vi "Read Offline Data.vi"(8 "Error In":errorcluster) -> (0 "Error Out":errorcluster)   [LabVIEW 2014, in "Aquisicao de Dados.lvlib"]
uses:
  Aquisicao de Dados.lvlib
  <vilib>/Waveform/WDTOps.llb/WDT Waveform Duration DBL.vi
  <vilib>/Waveform/WDTOps.llb/WDT Number of Waveform Samples DBL.vi
  <vilib>/measure/mascope.llb/Amplitude and Levels 1 chan.vi
  <vilib>/Waveform/WDTOps.llb/WDT Get Waveform Subset DBL.vi
  <vilib>/express/express analysis/Spectral/Block/exnSpectralBlock spectral measurements peak poly.vi
  <vilib>/express/express analysis/Spectral/Block/exnSpectralBlock spectral measurements peak WFM.vi
  <vilib>/express/express analysis/Spectral/XNode/ExpressSpectralMeasurementsBlockNode.xnode
  <vilib>/measure/NI_MAPro.lvlib
panel:
  out "Espectro Janelado":cluster{"f0":dbl, "df":dbl, "magnitude":dbl[]}(graph)
  in  "Duração":dbl(slide) scale=0.0..5.0
  in  "T inicial":dbl(slide) scale=0.0..5.0
  out "Frequência Fundamental":dbl
  out "Mulher":bool
  out "Homem":bool
  out "Canal 0":waveform(dbl)(graph)
  out "Resolução de Frequência":dbl
  out "Frequência Associada":dbl
  out "Maior Amplitude":dbl
  out "Período Amostral (s)":dbl
  out "Frequência Amostral (Hz)":dbl
  out "Número Amostral":dbl
  out "Amplitude do Sinal (%)":dbl
  out "Espectro do Canal 0":cluster{"f0":dbl, "df":dbl, "magnitude":dbl[]}(graph)
  out "Espectro do Canal 1":cluster{"f0":dbl, "df":dbl, "magnitude":dbl[]}(graph)
  out "Resolução de Frequência":dbl
  out "Frequência Associada":dbl
  out "Maior Amplitude":dbl
  out "Período Amostral (s)":dbl
  out "Frequência Amostral (Hz)":dbl
  out "Número Amostral":dbl
  out "Amplitude do Sinal (%)":dbl
  out "Canal 1":waveform(dbl)(graph)
  # "Dados do Sinal do Canal 0"
  # "Dados do Sinal do Canal 1"
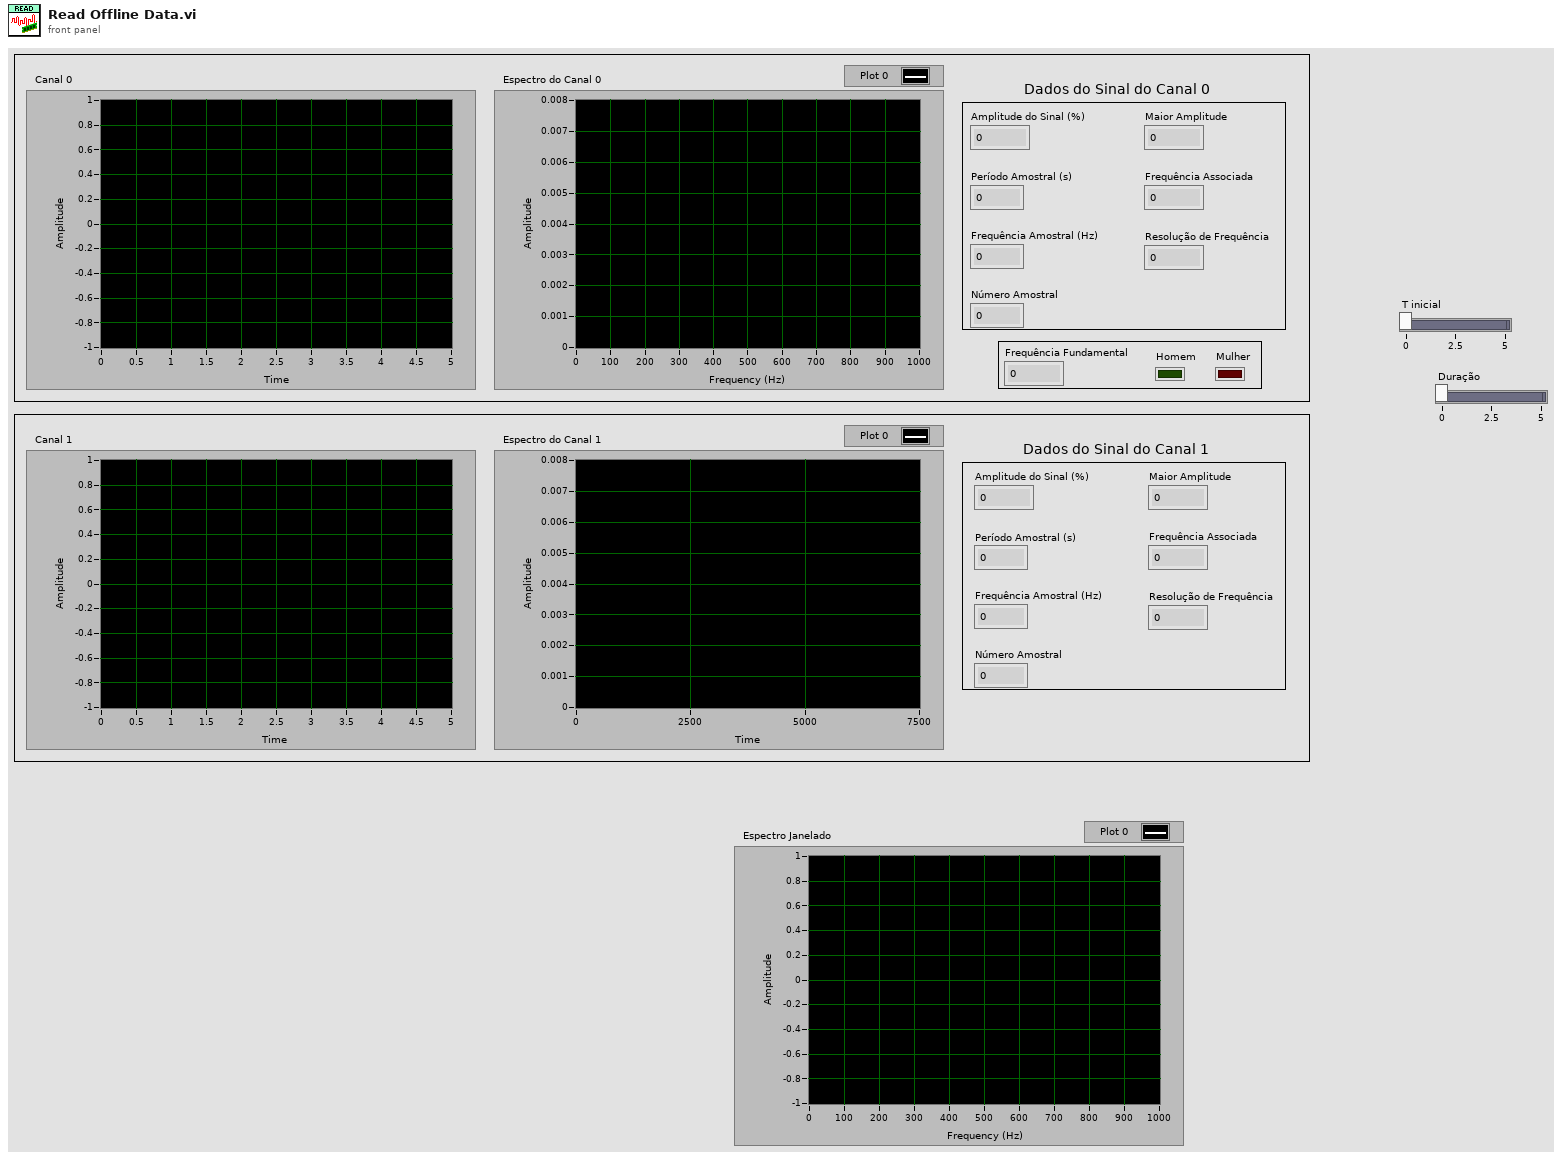
[diagram p1: front panel]
types:
  T1 = enum32{".WAV File", "LTSpice Simulation", "Microphone", "MultiSim Simulation", "Serial Port"}
  T2 = typedef "Aquisicao de Dados.lvlib/_ACC_DATA_ Config DAta State.ctl" = cluster{"_RAW_ Traces":cluster{"Trace Name":string, "Trace Type":string, "Trace Raw Data":dbl[], "Trace Waveform":waveform(dbl)}[], "_WAV_ Traces":waveform(dbl)[], "_MIC_ Config":cluster{"task ID":T3, "Data Chunk Size":i32, "Num Channels":i32, "Resolution":i32, "Sampling Frequency":dbl, "device ID":u32, "Num Chunks":i32}, "_LVM_ Traces":cluster{"Trace Name":string, "Trace Type":string, "Trace Raw Data":dbl[], "Trace Waveform":waveform(dbl)}[]}
  T3 = typedef "Sound Input Task ID.ctl" = u32
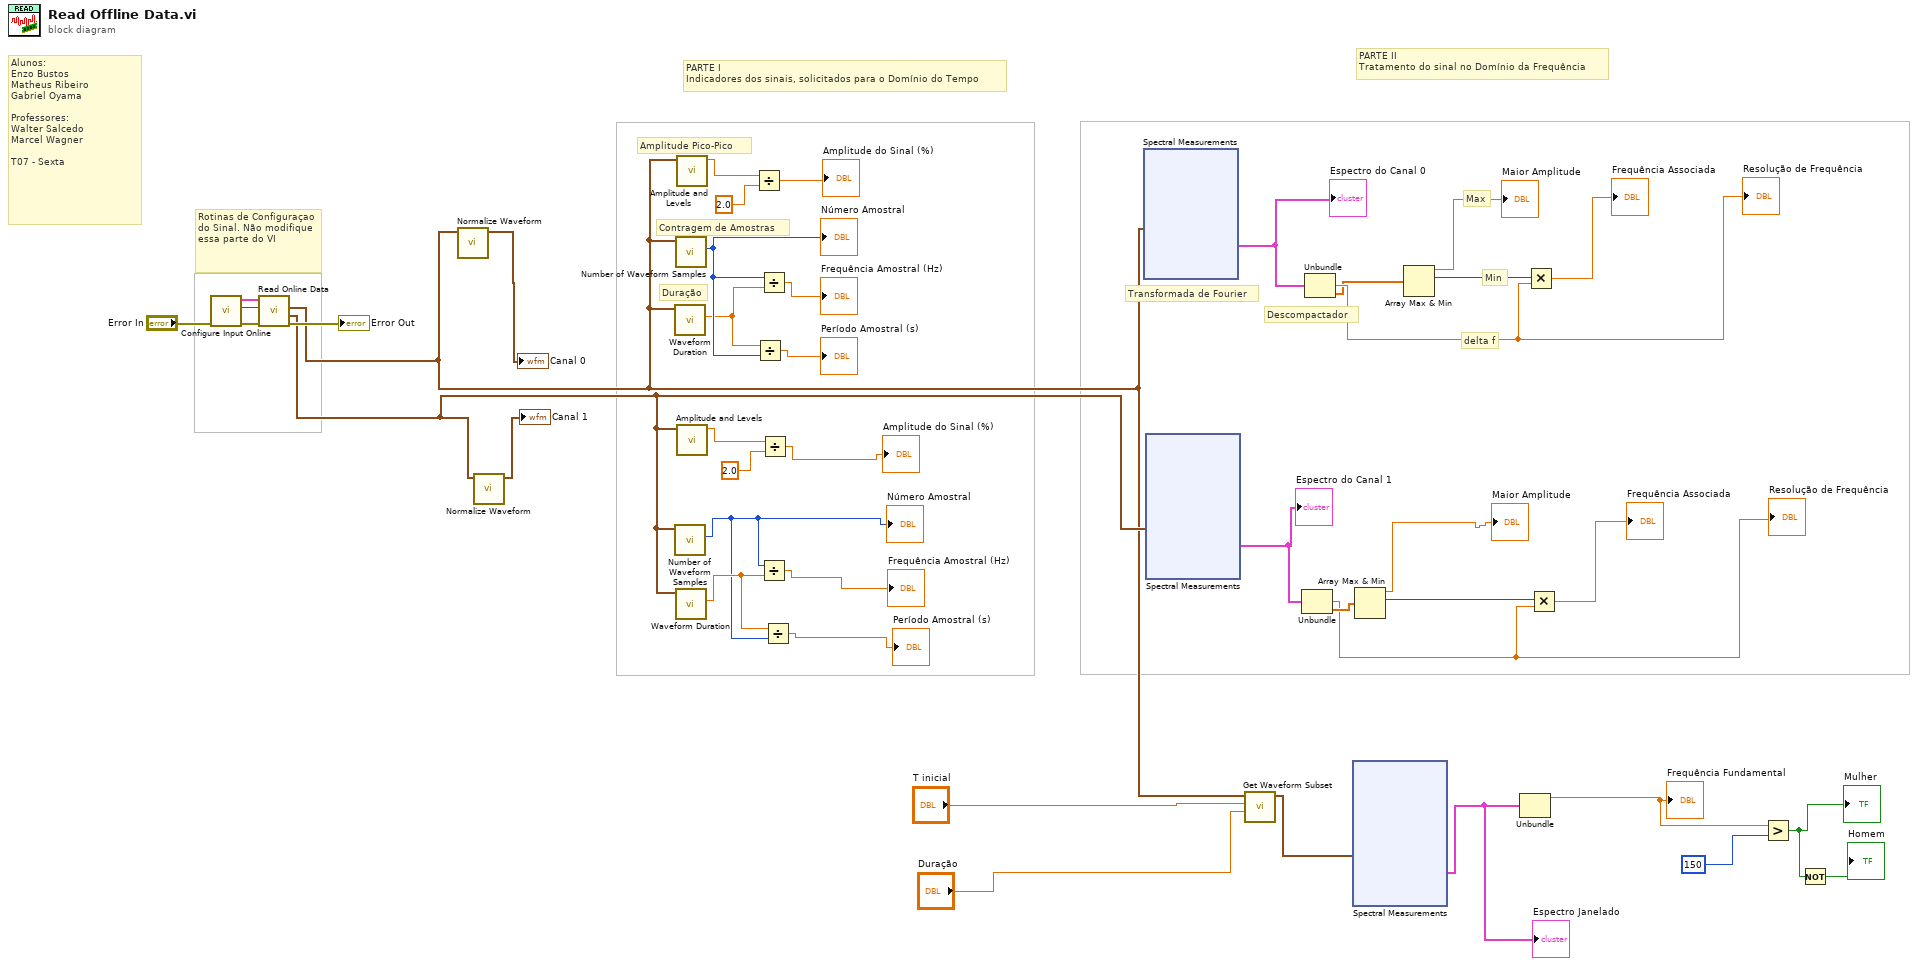
[diagram p0: block diagram]
diagram:
  # "Alunos:\nEnzo Bustos\nMatheus Ribeiro\nGabriel Oyama\n\nProfessores:\nWalter Salcedo\nMarcel Wagner\n\nT07 - Sexta"
  # "delta f"
  # "Min"
  # "Max"
  # "Descompactador"
  # "Transformada de Fourier"
  # "Duração"
  # "Contragem de Amostras"
  # "Amplitude Pico-Pico"
  # "PARTE II\nTratamento do sinal no Domínio da Frequência"
  # "PARTE I\nIndicadores dos sinais, solicitados para o Domínio do Tempo"
  # "Rotinas de Configuraçao do Sinal. Não modifique essa parte do VI"
  n1 = call "Configure Input Online.vi"("Error In"="Error In") -> ("Error Out"=w43:errorcluster, "Metodo de Entrada"=w41:T1, "Config Out"=w39:T2)  [unwired: 8 in]
  n2 = call "Read Online Data.vi"("Error In"=w43, "Metodo de Entrada"=w41, "Config Out"=w39) -> ("Error Out"=→"Error Out":errorcluster, "Channel 1"=w9:waveform(dbl), "Channel 0"=w6:waveform(dbl))  [unwired: 6 in]
  n3 = call <vilib>:"Normalize Waveform.vi"("waveform in"=w6) -> ("normalized waveform"=→"Canal 0":waveform(dbl))  [unwired: 7 in, 3 out]
  n4 = call <vilib>:"Normalize Waveform.vi"("waveform in"=w9) -> ("normalized waveform"=→"Canal 1":waveform(dbl))  [unwired: 7 in, 3 out]
  n5 = call-poly <vilib>:"Waveform Duration.vi"("waveform in"=w6) -> ("duration"=w32:dbl)  [unwired: 8 in, 2 out]
  n6 = call-poly <vilib>:"Number of Waveform Samples.vi"("waveform in"=w9) -> ("number of samples"=w22:i32)  [unwired: 8 in, 2 out]
  "Número Amostral" <- w22
  n7 = call-poly <vilib>:"Number of Waveform Samples.vi"("waveform in"=w6) -> ("number of samples"=w33:i32)  [unwired: 8 in, 2 out]
  "Número Amostral" <- w33
  n8 = call-poly <vilib>:"Waveform Duration.vi"("waveform in"=w9) -> ("duration"=w29:dbl)  [unwired: 8 in, 2 out]
  n9 = call-poly <vilib>:"Amplitude and Levels.vi"("signal in"=w6) -> ("amplitude"=w37:dbl)  [unwired: 7 in, 3 out]
  n10 = call-poly <vilib>:"Amplitude and Levels.vi"("signal in"=w9) -> ("amplitude"=w35:dbl)  [unwired: 7 in, 3 out]
  n11 = Divide(x=w37, y=2.0) -> (x/y=→"Amplitude do Sinal (%)":dbl)
  n12 = Divide(x=w32, y=w33) -> (x/y=→"Período Amostral (s)":dbl)
  n13 = Divide(x=w33, y=w32) -> (x/y=→"Frequência Amostral (Hz)":dbl)
  n14 = Divide(x=w22, y=w29) -> (x/y=→"Frequência Amostral (Hz)":dbl)
  n15 = Divide(x=w35, y=2.0) -> (x/y=→"Amplitude do Sinal (%)":dbl)
  n16 = Divide(x=w29, y=w22) -> (x/y=→"Período Amostral (s)":dbl)
  n17 = xnode "Spectral Measurements"("Signals"=w6) -> ("FFT - (Peak)"=w7:cluster{"f0":dbl, "df":dbl, "magnitude":dbl[]})  [unwired: 1 in, 2 out]
  "Espectro do Canal 0" <- w7
  n18 = xnode "Spectral Measurements"("Signals"=w9) -> ("FFT - (Peak)"=w26:cluster{"f0":dbl, "df":dbl, "magnitude":dbl[]})  [unwired: 1 in, 2 out]
  "Espectro do Canal 1" <- w26
  n19 = call-poly <vilib>:"Get Waveform Subset.vi"("duration"="Duração", "start samples/time"="T inicial", "waveform in"=w6) -> ("waveform out"=w4:waveform(dbl))  [unwired: 3 in, 3 out]
  n20 = Unbundle(w26) -> ("df"=w19:dbl, "magnitude"=w25:dbl[])  [unwired: 1 out]
  "Resolução de Frequência" <- w19
  n21 = Unbundle(w7) -> ("df"=w24:dbl, "magnitude"=w10:dbl[])  [unwired: 1 out]
  "Resolução de Frequência" <- w24
  n22 = xnode "Spectral Measurements"("Signals"=w4) -> ("FFT - (Peak)"=w2:cluster{"f0":dbl, "df":dbl, "magnitude":dbl[]})  [unwired: 1 in, 2 out]
  "Espectro Janelado" <- w2
  n23 = Array Max & Min(array=w25) -> (max value=→"Maior Amplitude":dbl, max index (indices)=w27:i32)  [unwired: 2 out]
  n24 = Array Max & Min(array=w10) -> (max value=→"Maior Amplitude":dbl, max index (indices)=w28:i32)  [unwired: 2 out]
  n25 = Unbundle(w2) -> ("f0"=w3:dbl)  [unwired: 2 out]
  "Frequência Fundamental" <- w3
  n26 = Multiply(x=w28, y=w24) -> (x*y=→"Frequência Associada":dbl)
  n27 = Multiply(x=w27, y=w19) -> (x*y=→"Frequência Associada":dbl)
  n28 = Greater?(x=w3, y=150) -> (0:w14:bool)
  "Mulher" <- w14
  n29 = Not(x=w14) -> (.not. x?=→"Homem":bool)
